vi "Get workfile.vi"(7 "Serial Port":refnum<visa-resource-name>) -> (1 "Serial Port":refnum<visa-resource-name>, 2 "On/Off status":T1, 3 "Workfile":T2 {"Purge B Off Time" format="%.2f"; "Purge B On Time" format="%.2f"; "Purge A Off Time" format="%.2f"; "Purge A On Time" format="%.2f"; "Det. B Time" format="%.2f"; "Det. A Time" format="%.2f"; "Final Time B" format="%.2f"; "Rate B" format="%.1f"; "Final Time A" format="%.2f"; "Rate A" format="%.1f"; "Final Time" format="%.2f"; "Rate" format="%.1f"; "Initial Time" format="%.2f"; "Equib Time" format="%.2f"})   [LabVIEW 2012]
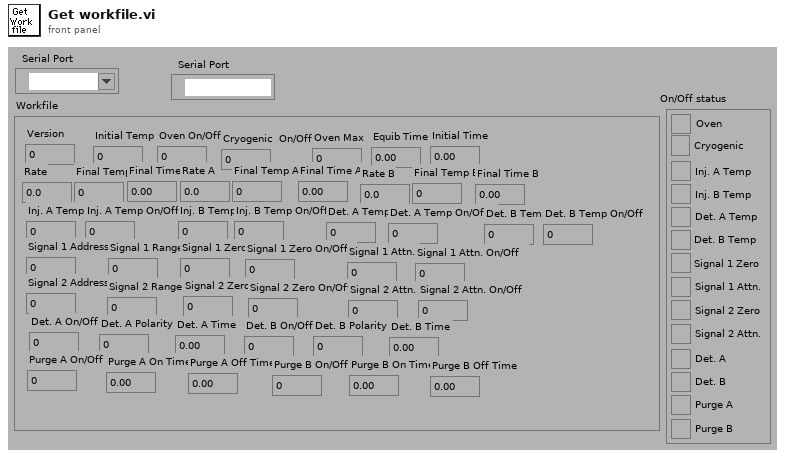
[diagram p1: front panel]
types:
  T1 = cluster{"Oven":bool, "Cryogenic":bool, "Inj. A Temp":bool, "Inj. B Temp":bool, "Det. A Temp":bool, "Det. B Temp":bool, "Signal 1 Zero":bool, "Signal 1 Attn.":bool, "Signal 2 Zero":bool, "Signal 2 Attn.":bool, "Det. A":bool, "Det. B":bool, "Purge A":bool, "Purge B":bool}
  T2 = cluster{"Version":sgl, "Initial Temp":sgl, "Oven On/Off":sgl, "Cryogenic  On/Off":sgl, "Oven Max":sgl, "Equib Time":sgl, "Initial Time":sgl, "Rate":dbl, "Final Temp":dbl, "Final Time":dbl, "Rate A":dbl, "Final Temp A":dbl, "Final Time A":dbl, "Rate B":dbl, "Final Temp B":dbl, "Final Time B":dbl, "Inj. A Temp":dbl, "Inj. A Temp On/Off":dbl, "Inj. B Temp":dbl, "Inj. B Temp On/Off":dbl, "Det. A Temp":dbl, "Det. A Temp On/Off":dbl, "Det. B Temp":dbl, "Det. B Temp On/Off":dbl, "Signal 1 Address":dbl, "Signal 1 Range":dbl, "Signal 1 Zero":dbl, "Signal 1 Zero On/Off":dbl, "Signal 1 Attn.":dbl, "Signal 1 Attn. On/Off":dbl, "Signal 2 Address":dbl, "Signal 2 Range":dbl, "Signal 2 Zero":dbl, "Signal 2 Zero On/Off":dbl, "Signal 2 Attn.":dbl, "Signal 2 Attn. On/Off":dbl, "Det. A On/Off":dbl, "Det. A Polarity":dbl, "Det. A Time":dbl, "Det. B On/Off":dbl, "Det. B Polarity":dbl, "Det. B Time":dbl, "Purge A On/Off":dbl, "Purge A On Time":dbl, "Purge A Off Time":dbl, "Purge B On/Off":dbl, "Purge B On Time":dbl, "Purge B Off Time":dbl}
  T3 = cluster{"[0]":dbl, "[1]":dbl, "[2]":dbl, "[3]":dbl, "[4]":dbl, "[5]":dbl, "[6]":dbl, "[7]":dbl, "[8]":dbl, "[9]":dbl, "[10]":dbl, "[11]":dbl, "[12]":dbl, "[13]":dbl, "[14]":dbl, "[15]":dbl, "[16]":dbl, "[17]":dbl, "[18]":dbl, "[19]":dbl, "[20]":dbl, "[21]":dbl, "[22]":dbl, "[23]":dbl, "[24]":dbl, "[25]":dbl, "[26]":dbl, "[27]":dbl, "[28]":dbl, "[29]":dbl, "[30]":dbl, "[31]":dbl, "[32]":dbl, "[33]":dbl, "[34]":dbl, "[35]":dbl, "[36]":dbl, "[37]":dbl, "[38]":dbl, "[39]":dbl, "[40]":dbl, "[41]":dbl, "[42]":dbl, "[43]":dbl, "[44]":dbl, "[45]":dbl, "[46]":dbl, "[47]":dbl}
  T4 = cluster{"[0]":bool, "[1]":bool, "[2]":bool, "[3]":bool, "[4]":bool, "[5]":bool, "[6]":bool, "[7]":bool, "[8]":bool, "[9]":bool, "[10]":bool, "[11]":bool, "[12]":bool, "[13]":bool}
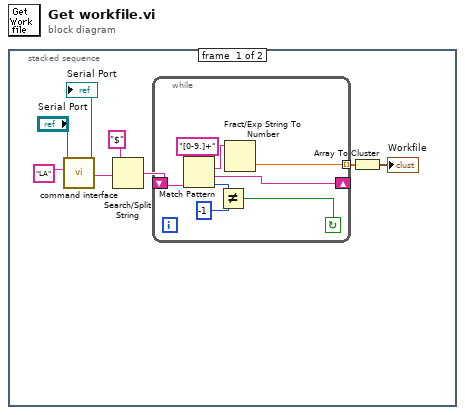
[diagram p0: block diagram]
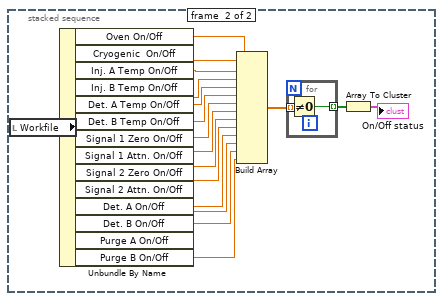
[diagram p2: hidden frame]
diagram:
  n1 = stacked-sequence {
    frame #0 {
      n2 = call "command interface.vi"("command"="LA", "Serial Port"="Serial Port") -> ("response"=w4:string, "Serial Port"=→"Serial Port":refnum<visa-resource-name>)  [unwired: 5 in, 2 out]
      n3 = Search/Split String(string=w4, search string/char (-)="$") -> (match + rest of string=w6:string)  [unwired: 1 in, 2 out]
      n4 = while {
        tunnel: [w12] -> w5 mode=indexing
        shift-left: w6 -> [w16]
        shift-right: [w13] -> _
        stop <- w10 continue-if-true
        n5 = Match Pattern(string=w16, regular expression="[0-9.]+") -> (match substring=w14:string, after substring=w13:string, offset past match=w11:i32)  [unwired: 1 in, 1 out]
        n6 = Not Equal?(x=w11, y=-1) -> (x != y?=w10:bool)
        n7 = Fract/Exp String To Number(string=w14) -> (number=w12:dbl)  [unwired: 3 in, 1 out]
      }
      n8 = Array To Cluster(array=w5) -> (cluster=→"Workfile":T3)
    }
    frame #1 {
      n9 = local read "Workfile"() -> (w34:T2)
      n10 = Unbundle By Name(w34) -> ("Oven On/Off"=w33:sgl, "Cryogenic  On/Off"=w32:sgl, "Inj. A Temp On/Off"=w31:dbl, "Inj. B Temp On/Off"=w30:dbl, "Det. A Temp On/Off"=w29:dbl, "Det. B Temp On/Off"=w28:dbl, "Signal 1 Zero On/Off"=w27:dbl, "Signal 1 Attn. On/Off"=w26:dbl, "Signal 2 Zero On/Off"=w25:dbl, "Signal 2 Attn. On/Off"=w24:dbl, "Det. A On/Off"=w23:dbl, "Det. B On/Off"=w22:dbl, "Purge A On/Off"=w21:dbl, "Purge B On/Off"=w20:dbl)
      n11 = Build Array(w33, w32, w31, w30, w29, w28, w27, w26, w25, w24, w23, w22, w21, w20) -> (w19:dbl[])
      n12 = for {
        tunnel: w19 -> [w36] mode=indexing
        tunnel: [w35] -> w18 mode=indexing
        n13 = Not Equal To 0?(x=w36) -> (x != 0?=w35:bool)
      }
      n14 = Array To Cluster(array=w18) -> (cluster=→"On/Off status":T4)
    }
  }
